vi "Array of Python Strings to Python List.vi"(8 "error in (no error)":errorcluster, 10 "Array of Python Strings":string[](array[string])) -> (0 "error out":errorcluster, 2 "Python List":string)   [LabVIEW 2020, in "jki_python_data_tools.lvlib"]
uses:
  jki_python_data_tools.lvlib
  <userlib>/_OpenG.lib/string/string.llb/openg_string.lvlib
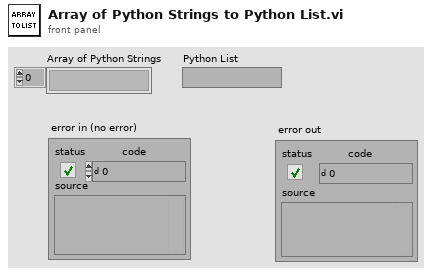
[diagram p1: front panel]
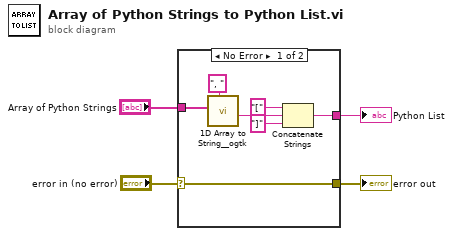
[diagram p0: block diagram]
diagram:
  n1 = case shown="No Error" "error in (no error)" {
    selector: "error in (no error)" -> [w5 w12]
    tunnel: [w11 _] -> w4
    tunnel: "Array of Python Strings" -> [w10 _]
    tunnel: [w5 w12] -> w1
    frame No Error {
      n2 = call <userlib>:"1D Array to String__ogtk.vi"("delimiter (Tab)"=", ", "Array of Strings"=w10) -> ("delimited string"=w7:string)  [unwired: 9 in]
      n3 = Concatenate Strings("[" ("string"), w7, "]" ("string")) -> (w11:string)
    }
    frame Error {
    }
  }
  "Python List" <- w4
  "error out" <- w1
